vi "DOnames.vi"() -> (3 "DIO Channel":T1)   [LabVIEW 2015]
doc: "Uses this constant to define channels and names for digital outputs"
uses:
  <vilib>/Rock Robotics/SystemInterfaces/DIO/FPGA_DIOChannel.ctl
  DOs.ctl
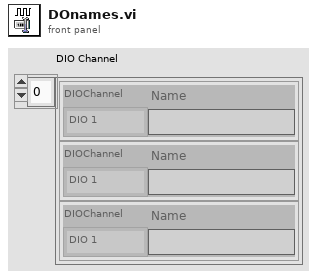
[diagram p1: front panel]
types:
  T1 = typedef "DOs.ctl" = cluster{"DIOChannel":T2, "Name":string}[]
  T2 = typedef "FPGA_DIOChannel.ctl" = enum8{"DIO 1", "DIO 2", "DIO 3", "DIO 4", "DIO 5", "DIO 6", "DIO 7", "DIO 8", "DIO 9", "DIO 10", "DIO 11", "DIO 12", "DIO 13", "DIO 14", "Invalid"}
  T3 = typedef "DOs.ctl" = cluster{"DIOChannel":T4, "Name":string}[]
  T4 = typedef "FPGA_DIOChannel.ctl" = enum8{"DIO 0", "DIO 1", "DIO 2", "DIO 3", "DIO 4", "DIO 5", "DIO 6", "DIO 7", "DIO 8", "DIO 9", "DIO MXP 0", "DIO MXP 1", "DIO MXP 2", "DIO MXP 3", "DIO MXP 4", "DIO MXP 5", "DIO MXP 6", "DIO MXP 7", "DIO MXP 8", "DIO MXP 9", "DIO MXP 10", "DIO MXP 11", "DIO MXP 12", "DIO MXP 13", "DIO MXP 14", "DIO MXP 15", "Invalid"}
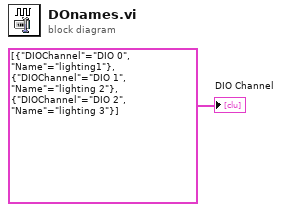
[diagram p0: block diagram]
diagram:
  "DIO Channel" <- T3 [{"DIOChannel"=enum."DIO 0", "Name"="lighting1"}, {"DIOChannel"=enum."DIO 1", "Name"="lighting 2"}, {"DIOChannel"=enum."DIO 2", "Name"="lighting 3"}] ("DIO Channel 2")
